vi "AddPvtValueToIpmBuffer.vi"(4 "error in (no error)":errorcluster, 5 "PVT value":T1, 7 "axis in":cluster{"keyHandle":u32, "nodeId":u16}={"keyHandle"=0, "nodeId"=1}) -> (0 "error out":errorcluster, 3 "axis out":cluster{"keyHandle":u32, "nodeId":u16}={"keyHandle"=0, "nodeId"=1})   [LabVIEW 2017, in "maxonEPOS.lvlib"]
doc: "<B>AddPvtValueToIpmBuffer</B> writes a new PVT reference point to the device."
uses:
  Examples/maxonEPOS.lvlib
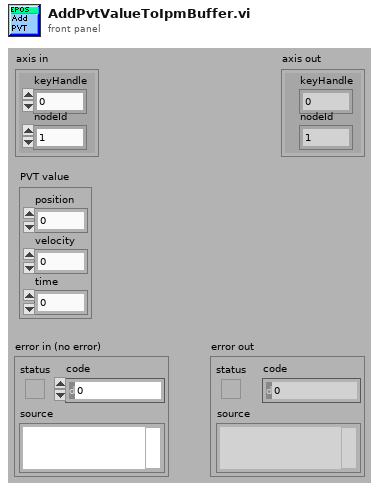
[diagram p1: front panel]
types:
  T1 = cluster{"position":i32, "velocity":i32, "time":u8}
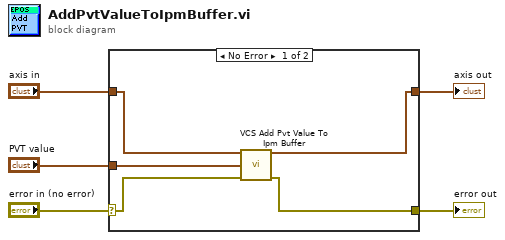
[diagram p0: block diagram]
diagram:
  n1 = case shown="No Error" "error in (no error)" {
    selector: "error in (no error)" -> [w10 w12]
    tunnel: [w9 w12] -> w4
    tunnel: [w8 w11] -> w3
    tunnel: "axis in" -> [w6 w11]
    tunnel: "PVT value" -> [w7 _]
    frame No Error {
      n2 = call "VCS Add Pvt Value To Ipm Buffer.vi"("axis in"=w6, "PVT value"=w7, "error in (no error)"=w10) -> ("axis out"=w8:cluster{"keyHandle":u32, "nodeId":u16}, "error out"=w9:errorcluster)  [unwired: 11 in]
    }
    frame Error {
    }
  }
  "error out" <- w4
  "axis out" <- w3
